vi "Odbior danych z PC .vi"(8 "error in (no error)":errorcluster, 11 "connection ID":refnum<k16>) -> (0 "error out":errorcluster, 1 "jazda":T1[](array[typedef]) {"type" items=["CAN Data", "CAN Remote"]; "identifier" format="%.0x"}, 2 "konf":T1 {"type" items=["CAN Data", "CAN Remote"]; "identifier" format="%.0x"}, 3 "connection ID out":refnum<k16>)   [LabVIEW 2015]
uses:
  <vilib>/RioEmbeddedCAN/RioEmbeddedCAN.llb/CANFrameControl.ctl
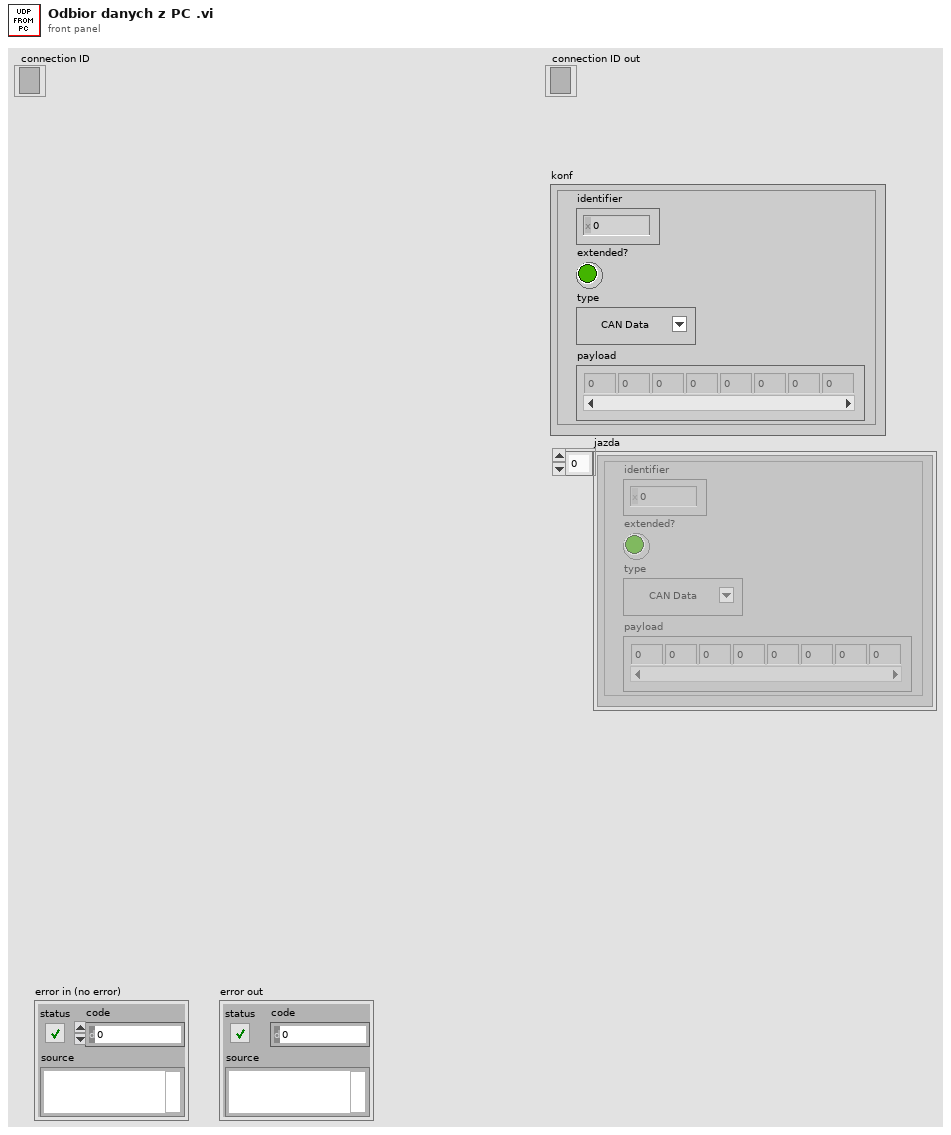
[diagram p1: front panel]
types:
  T1 = typedef "CANFrameControl.ctl" = cluster{"identifier":u32, "extended?":bool, "type":u8, "payload":u8[]}
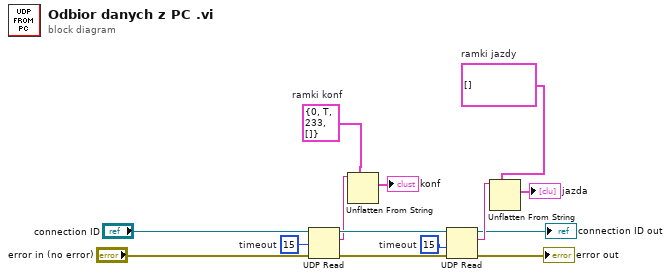
[diagram p0: block diagram]
diagram:
  w3 = 15  # timeout
  w4 = 15  # timeout
  w13 = T1[] []  # ramki jazdy
  w14 = T1 {"identifier"=0, "extended?"=TRUE, "type"=233, "payload"=[]}  # ramki konf
  n1 = UDP Read(connection ID="connection ID", timeout ms (25000)=w3, 8:"error in (no error)") -> (data out=w7:string, error out=w10:errorcluster, 3:w8:refnum<k16>)  [unwired: 1 in, 2 out]
  n2 = Unflatten From String(type=w14, binary string=w7) -> (value=→"konf":T1)  [unwired: 3 in, 2 out]
  n3 = UDP Read(connection ID=w8, timeout ms (25000)=w4, 8:w10) -> (data out=w6:string, error out=→"error out":errorcluster, 3:→"connection ID out":refnum<k16>)  [unwired: 1 in, 2 out]
  n4 = Unflatten From String(type=w13, binary string=w6) -> (value=→"jazda":T1[])  [unwired: 3 in, 2 out]
